vi "test.vi"() -> ()   [LabVIEW 2014]
panel:
  out "out2":string
  out "out1":string
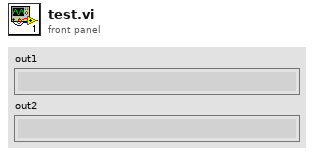
[diagram p1: front panel]
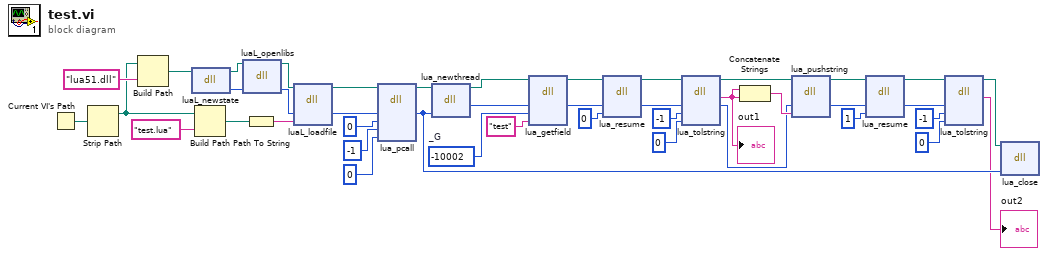
[diagram p0: block diagram]
diagram:
  w24 = -10002  # _G
  n1 = Current VI's Path() -> (path=w42:path)
  n2 = Strip Path(path=w42) -> (stripped path=w33:path)  [unwired: 1 out]
  n3 = Build Path(base path=w33, name or relative path="lua51.dll") -> (appended path=w40:path)
  n4 = dll-call lib="D:/Desktop/lua51.dll" fn="luaL_newstate"(path in=w40) -> (path out=w38:path, "L"=w39:u64)  [unwired: 2 in, 1 out]
  n5 = Build Path(base path=w33, name or relative path="test.lua") -> (appended path=w31:path)
  n6 = dll-call lib="D:/Desktop/lua51.dll" fn="luaL_openlibs"(path in=w38, "L"=w39) -> (path out=w37:path, "L"=w35:u64)  [unwired: 3 in, 1 out]
  n7 = Path To String(path=w31) -> (string=w30:string)
  n8 = dll-call lib="D:/Desktop/lua51.dll" fn="luaL_loadfile"(path in=w37, "L"=w35, "path"=w30) -> (path out=w36:path, "L"=w34:u64)  [unwired: 4 in, 1 out]
  n9 = dll-call lib="D:/Desktop/lua51.dll" fn="lua_pcall"(path in=w36, "L"=w34, "nargs"=0 ("nresults"), "nresults"=-1, "errfunc"=0) -> (path out=w26:path, "L"=w14:u64)  [unwired: 6 in, 1 out]
  n10 = dll-call lib="D:/Desktop/lua51.dll" fn="lua_newthread"(path in=w26, "L"=w14) -> (path out=w25:path, "thread"=w20:u64)  [unwired: 3 in, 1 out]
  n11 = dll-call lib="D:/Desktop/lua51.dll" fn="lua_getfield"(path in=w25, "L"=w20, "idx"=w24, "key"="test") -> (path out=w21:path, "L"=w19:u64)  [unwired: 5 in, 1 out]
  n12 = dll-call lib="D:/Desktop/lua51.dll" fn="lua_resume"(path in=w21, "L"=w19, "narg"=0) -> (path out=w15:path, "L"=w18:u64)  [unwired: 4 in, 1 out]
  n13 = dll-call lib="D:/Desktop/lua51.dll" fn="lua_tolstring"(path in=w15, "L"=w18, "idx"=-1, "len"=0) -> (path out=w12:path, "str"=w9:string, "L"=w1:u64)  [unwired: 4 in, 1 out]
  "out1" <- w9
  n14 = Concatenate Strings(w9, w9) -> (w8:string)
  n15 = dll-call lib="D:/Desktop/lua51.dll" fn="lua_pushstring"(path in=w12, "L"=w1, "str"=w8) -> (path out=w11:path, "L"=w10:u64)  [unwired: 4 in, 1 out]
  n16 = dll-call lib="D:/Desktop/lua51.dll" fn="lua_resume"(path in=w11, "L"=w10, "narg"=1) -> (path out=w4:path, "L"=w7:u64)  [unwired: 4 in, 1 out]
  n17 = dll-call lib="D:/Desktop/lua51.dll" fn="lua_tolstring"(path in=w4, "L"=w7, "idx"=-1, "len"=0) -> (path out=w3:path, "str"=→"out2":string)  [unwired: 5 in, 1 out]
  n18 = dll-call lib="D:/Desktop/lua51.dll" fn="lua_close"(path in=w3, "L"=w14) -> ()  [unwired: 4 in, 2 out]
